vi "Read data depth.vi"(4 "Error In":errorcluster, 7 "Set Data Buffer Depth in":refnum<class "Remote Access Commands_Set Data Buffer Depth.lvclass">) -> (0 "Error Out":errorcluster, 2 "data depth":i32, 3 "Set Data Buffer Depth out":refnum<class "Remote Access Commands_Set Data Buffer Depth.lvclass">)   [LabVIEW 2015, in "Startup Processes.lvlib" / "Remote Access Commands_Set Data Buffer Depth.lvclass"]
uses:
  Remote Access Commands_Set Data Buffer Depth.lvclass
  Remote Access Commands_Set Data Buffer Depth.lvclass/Remote Access Commands_Set Data Buffer Depth.ctl
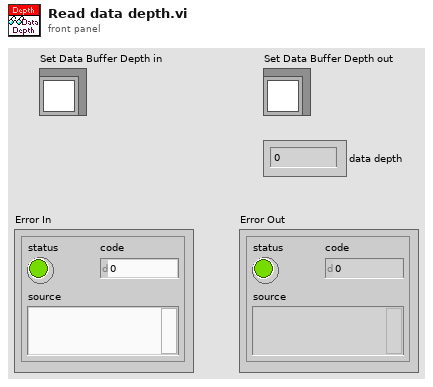
[diagram p1: front panel]
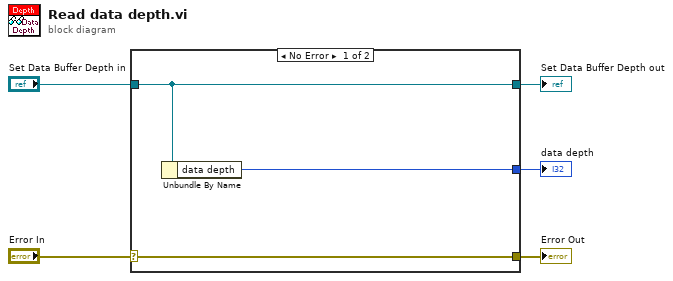
[diagram p0: block diagram]
diagram:
  n1 = case shown="No Error" "Error In" {
    selector: "Error In" -> [w8 w9]
    tunnel: [w8 w9] -> w4
    tunnel: [w7 w10] -> w2
    tunnel: "Set Data Buffer Depth in" -> [w7 w10]
    tunnel: [w6 _] -> w1
    frame No Error {
      n2 = Unbundle By Name(w7) -> ("data depth"=w6:i32)
    }
    frame Error {
    }
  }
  "Error Out" <- w4
  "Set Data Buffer Depth out" <- w2
  "data depth" <- w1
